vi "GEMM(CuLab).vi"() -> ()   [LabVIEW 2020]
uses:
  13ac56ee-d342-4fc9-916d-ee8b581d680f.vi
  e733ec95-1f17-4a92-a93c-f13053a3e0ea.vi
  <vilib>/Analysis/baseanly.llb/Mean (DBL).vi
  <vilib>/Utility/High Resolution Relative Seconds.vi
  <vilib>/Ngene/CuLab - GPU Accelerated Toolkit/Toolkit/Low_Level/Tensor_Classes/T_Children/T2D/T2D_Children/T2D_SGL/Create.vi
  <vilib>/Ngene/CuLab - GPU Accelerated Toolkit/Toolkit/Low_Level/Tensor_Classes/T_Children/T2D/T2D_Children/T2D_SGL/Push.vi
  <vilib>/Ngene/CuLab - GPU Accelerated Toolkit/Toolkit/API/Linear Algebra/BLAS3/gemm/CU_gemm/CU_Sgemm.vi
  <vilib>/Ngene/CuLab - GPU Accelerated Toolkit/Toolkit/Low_Level/Tensor_Classes/T_Children/T2D/T2D_Children/T2D_SGL/Pull_to_DVR.vi
  <vilib>/Utility/file.llb/Write Delimited Spreadsheet (string).vi
  <vilib>/Analysis/NI_AALBase.lvlib
  <vilib>/Ngene/CuLab - GPU Accelerated Toolkit/Toolkit/CuLab.lvlib
  <vilib>/Ngene/CuLab - GPU Accelerated Toolkit/Toolkit/Low_Level/Tensor_Classes/T_Children/T2D/T2D_Children/T2D_SGL/T2D_SGL.lvclass
panel:
  out "Results":dbl[](graph)=[0.09012666681276946, 0.10166666688746773, 0.4007333326929559, 1.2280399993566486, 4.011626665548344, 13.208833333677225, 104.1542199998124, 1369.7864866667564]
  out "error out":errorcluster
  in  "Benchmark Params":cluster{"Size":i32, "Iteration":i32}[](array[cluster])=[{"Size"=64, "Iteration"=20}, {"Size"=128, "Iteration"=20}, {"Size"=256, "Iteration"=20}, {"Size"=512, "Iteration"=20}, {"Size"=1024, "Iteration"=20}, {"Size"=2048, "Iteration"=20}, {"Size"=4096, "Iteration"=20}, {"Size"=8192, "Iteration"=20}]
  out "Results(ms)":dbl[](array[numeric])=[0.09012666681276946, 0.10166666688746773, 0.4007333326929559, 1.2280399993566486, 4.011626665548344, 13.208833333677225, 104.1542199998124, 1369.7864866667564] format="%.7f"
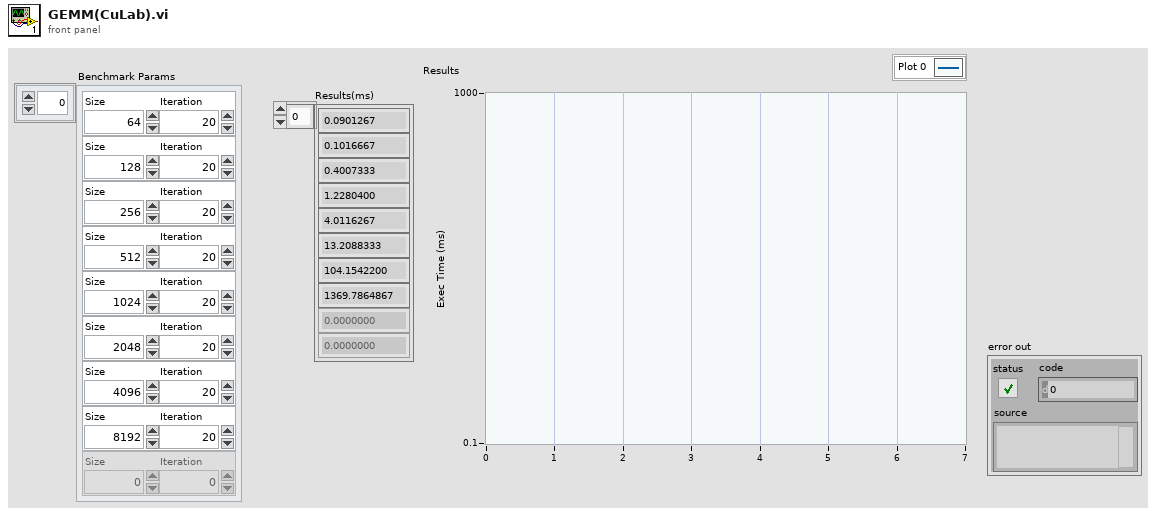
[diagram p1: front panel]
types:
  T1 = typedef "CuLab.lvlib/CuLab_Data_ref_2D_SGL.ctl" = refnum<data-value>
  T2 = typedef "CuLab.lvlib/Properties.ctl" = cluster{"Device ID":i32, "Name":string}
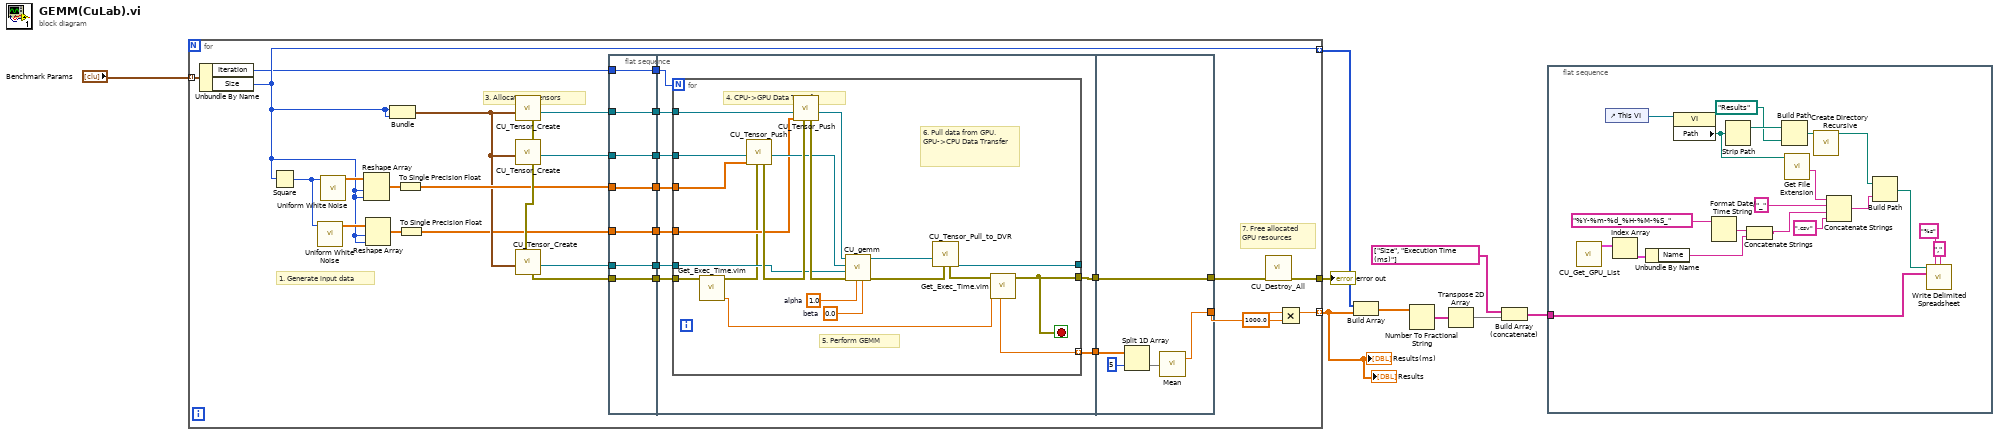
[diagram p0: block diagram]
diagram:
  n1 = for {
    tunnel: "Benchmark Params" -> [w35] mode=indexing
    tunnel: [w30] -> w3
    tunnel: [w11] -> w1 mode=indexing
    tunnel: [w17] -> w6 mode=indexing
    # "7. Free allocated \nGPU resources"
    # "3. Allocate 2D Tensors"
    # "1.\tGenerate input data"
    n2 = Unbundle By Name(w35) -> ("Iteration"=w12:i32, "Size"=w17:i32)
    n3 = Square(x=w17) -> (x^2=w29:i32)
    n4 = call <vilib>:"Uniform White Noise.vi"("samples"=w29) -> ("uniform white noise"=w33:dbl[])  [unwired: 9 in, 1 out]
    n5 = call <vilib>:"Uniform White Noise.vi"("samples"=w29) -> ("uniform white noise"=w34:dbl[])  [unwired: 9 in, 1 out]
    n6 = Reshape Array(w34, w17, w17) -> (w31:dbl[][])
    n7 = Reshape Array(w33, w17, w17) -> (w32:dbl[][])
    n8 = Bundle("Size"=w17, "Size"=w17) -> (w16:cluster{"Size":i32, "Size":i32})  [unwired: 1 in]
    n9 = To Single Precision Float(number=w31) -> (single precision float=w38:sgl[][])
    n10 = To Single Precision Float(number=w32) -> (single precision float=w13:sgl[][])
    n11 = call-poly <vilib>:"CU_Tensor_Create.vi"("T2D_Dims"=w16) -> ("T2D_SGL out"=w37:refnum<class "T2D_SGL.lvclass">, "error out"=w40:errorcluster)  [unwired: 9 in]
    n12 = call-poly <vilib>:"CU_Tensor_Create.vi"("error in (no error)"=w40, "T2D_Dims"=w16) -> ("T2D_SGL out"=w36:refnum<class "T2D_SGL.lvclass">, "error out"=w39:errorcluster)  [unwired: 8 in]
    n13 = call-poly <vilib>:"CU_Tensor_Create.vi"("error in (no error)"=w39, "T2D_Dims"=w16) -> ("T2D_SGL out"=w28:refnum<class "T2D_SGL.lvclass">, "error out"=w27:errorcluster)  [unwired: 8 in]
    n14 = flat-sequence {
      tunnel: w27 -> [w41]
      tunnel: w28 -> [w42]
      tunnel: w12 -> [w43]
      tunnel: w36 -> [w44]
      tunnel: w37 -> [w45]
      tunnel: w13 -> [w46]
      tunnel: w38 -> [w47]
      tunnel: [w47] -> w23
      tunnel: [w46] -> w22
      tunnel: [w45] -> w21
      tunnel: [w44] -> w20
      tunnel: [w43] -> w19
      tunnel: [w42] -> w18
      tunnel: [w41] -> w14
      tunnel: [w51] -> w24
      tunnel: w23 -> [w56]
      tunnel: w22 -> [w55]
      tunnel: w21 -> [w54]
      tunnel: w20 -> [w53]
      tunnel: w19 -> [w50]
      tunnel: w18 -> [w52]
      tunnel: [w49] -> w15
      tunnel: w14 -> [w48]
      tunnel: [w77] -> w25
      tunnel: [w81] -> w26
      tunnel: w24 -> [w81]
      tunnel: w15 -> [w80]
      frame #0 {
      }
      frame #1 {
        n15 = for {
          N: w50 -> [_]
          tunnel: w56 -> [w64]
          tunnel: w55 -> [w63]
          tunnel: w54 -> [w71]
          tunnel: w53 -> [w73]
          tunnel: w52 -> [w62]
          tunnel: [w67] -> _
          tunnel: [w65] -> w51
          tunnel: [w58] -> w49 mode=indexing
          tunnel: w48 -> [w57]
          stop <- w65 stop-if-true
          w75 = sgl 0.0  # beta
          w76 = sgl 1.0  # alpha
          # "6. Pull data from GPU.\nGPU->CPU Data Transfer"
          # "5. Perform GEMM"
          # "4. CPU->GPU Data Transfer"
          n16 = call "Get_Exec_Time.vim"("error in (no error)"=w57) -> ("T(n)"=w59:dbl, "error out"=w61:errorcluster)  [unwired: 6 in, 1 out]
          n17 = call-poly <vilib>:"CU_Tensor_Push.vi"("error in (no error)"=w61, "CPU_Data_2D_SGL"=w64, "T2D_SGL in"=w73) -> ("T2D_SGL out"=w66:refnum<class "T2D_SGL.lvclass">, "error out"=w72:errorcluster)  [unwired: 7 in]
          n18 = call-poly <vilib>:"CU_Tensor_Push.vi"("error in (no error)"=w72, "CPU_Data_2D_SGL"=w63, "T2D_SGL in"=w71) -> ("T2D_SGL out"=w68:refnum<class "T2D_SGL.lvclass">, "error out"=w69:errorcluster)  [unwired: 7 in]
          n19 = call-poly <vilib>:"CU_gemm.vi"("beta"=w75, "alpha"=w76, "error in (no error)"=w69, "C"=w62, "B"=w66, "A"=w68) -> ("error out"=w74:errorcluster, "C out"=w70:refnum<class "T2D_SGL.lvclass">)  [unwired: 4 in]
          n20 = call-poly <vilib>:"CU_Tensor_Pull_to_DVR.vi"("error in (no error)"=w74, "T2D_SGL in"=w70) -> ("Dest out"=w67:T1, "error out"=w60:errorcluster)  [unwired: 7 in, 1 out]
          n21 = call "Get_Exec_Time.vim"("T(n-1)"=w59, "error in (no error)"=w60) -> ("error out"=w65:errorcluster, "dT"=w58:dbl)  [unwired: 5 in, 1 out]
        }
      }
      frame #2 {
        n22 = Split 1D Array(array=w80, index=5) -> (second subarray=w78:dbl[])  [unwired: 1 out]
        n23 = call-poly <vilib>:"Mean.vi"("X"=w78) -> ("mean"=w77:dbl)  [unwired: 1 out]
      }
    }
    n24 = call <vilib>:"CU_Destroy_All.vi"("error in"=w26) -> ("error out"=w30:errorcluster)  [unwired: 10 in]
    n25 = Multiply(x=w25, y=1000.0) -> (x*y=w11:dbl)
  }
  "Results(ms)" <- w1
  "error out" <- w3
  "Results" <- w1
  n26 = Build Array(w6, w1) -> (w9:dbl[][])
  n27 = Number To Fractional String(number=w9) -> (F-format string=w8:string[][])  [unwired: 3 in]
  n28 = Transpose 2D Array(2D array=w8) -> (transposed array=w5:string[][])
  n29 = Build Array (concatenate)(string[] ["Size", "Execution Time (ms)"] ("element"), w5) -> (w2:string[][])
  n30 = flat-sequence {
    tunnel: w2 -> [w101]
    frame #0 {
      n31 = call <vilib>:"CU_Get_GPU_List.vi"() -> ("Devices"=w85:T2[])  [unwired: 10 in, 1 out]
      n32 = control-ref of="This VI"() -> (w95:refnum<vi>)
      n33 = Index Array(array=w85) -> (element=w84:T2)  [unwired: 1 in]
      n34 = Unbundle By Name(w84) -> ("Name"=w83:string)
      n35 = property class="VI"(reference=w95) -> ("Path"=w90:path)  [unwired: 1 in, 2 out]
      n36 = Format Date/Time String(time format string (%c)="%Y-%m-%d_%H-%M-%S_") -> (date/time string=w86:string)  [unwired: 2 in]
      n37 = Strip Path(path=w90) -> (stripped path=w94:path)  [unwired: 1 out]
      n38 = Concatenate Strings(w86, w83) -> (w82:string)
      n39 = Build Path(base path=w94, name or relative path=path "Results") -> (appended path=w93:path)
      n40 = call <vilib>:"Get File Extension.vi"("file"=w90) -> ("filename without extension"=w89:string)  [unwired: 6 in, 4 out]
      n41 = call <vilib>:"Create Directory Recursive.vi"("directory"=w93) -> ("directory copy"=w91:path)  [unwired: 4 in, 2 out]
      n42 = Concatenate Strings(w89, "_" ("string"), w82, ".csv" ("string")) -> (w99:string)
      n43 = Build Path(base path=w91, name or relative path=w99) -> (appended path=w100:path)
      n44 = call-poly <vilib>:"Write Delimited Spreadsheet.vi"("file path (dialog if empty)"=w100, "format (%s)"="%s", "2D data"=w101, "delimiter (\\t)"="," ("delimiter (\\t)")) -> ()  [unwired: 10 in, 2 out]
    }
  }
